vi "Pointer.Read (String).vi"(8 "error in (no error)":errorcluster, 10 "count":i32, 11 "pointer in":u64) -> (0 "error out":errorcluster, 2 "string out":string, 3 "pointer out":u64)   [LabVIEW 2016, in "VeriStand Data.lvlib"]
doc: "Reads a number of values, specified by <B>count</B>, from the provided <B>pointer</B>."
uses:
  VeriStand Data.lvlib
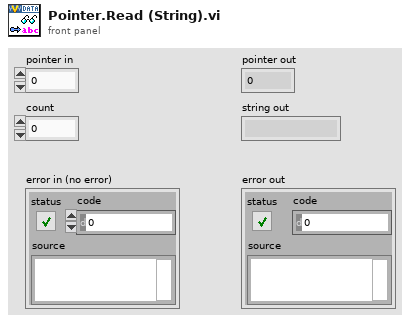
[diagram p1: front panel]
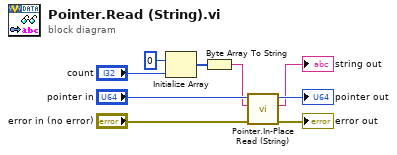
[diagram p0: block diagram]
diagram:
  n1 = Initialize Array(u8 0 ("element"), "count") -> (w2:u8[])
  n2 = Byte Array To String(unsigned byte array=w2) -> (string=w1:string)
  n3 = call "Pointer.In-Place Read (String).vi"("error in (no error)"="error in (no error)", "allocated string in"=w1, "pointer in"="pointer in") -> ("error out"=→"error out":errorcluster, "string out"=→"string out":string, "pointer out"=→"pointer out":u64)  [unwired: 6 in]
